vi "Path Keeper_User Find File.vi"(7 "Previous Path":path, 8 "error In":errorcluster, 9 "File(f)\nDirectory(t) In":bool, 11 "File / Directory Name In":string) -> (0 "error Out":errorcluster, 1 "Valid Item Out":bool, 3 "path Out":path)   [LabVIEW 2015]
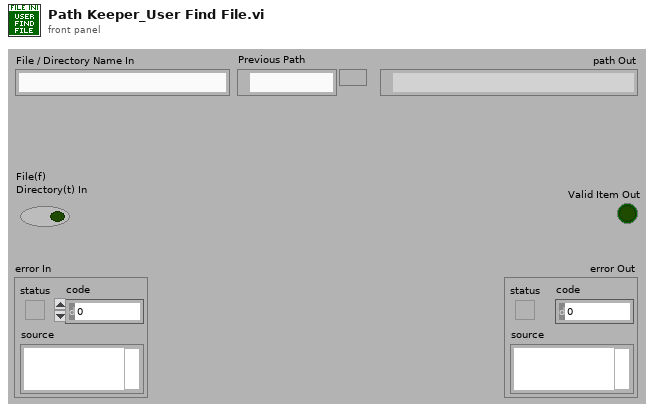
[diagram p1: front panel]
types:
  T1 = enum32{"existing file", "new file", "new or existing file", "existing dir", "new dir", "new or existing dir", "existing file (use LLBs)", "new file (use LLBs)", "new or existing file (use LLBs)", "new or existing file or directory (use LLBs)"}
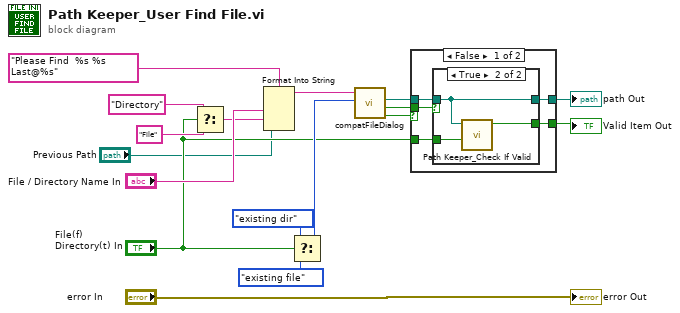
[diagram p0: block diagram]
diagram:
  n1 = Select(t="Directory" ("File / Directory Name In"), s="File(f)\nDirectory(t) In", f="File") -> (s? t:f=w6:string)
  n2 = Format Into String(format string="Please Find  %s %s Last@%s", "File / Directory Name In", w6, "Previous Path") -> (resulting string=w5:string)  [unwired: 2 in, 1 out]
  n3 = Select(t=T1."existing dir" ("select mode (2)"), s="File(f)\nDirectory(t) In", f=T1."existing file" ("select mode (2)")) -> (s? t:f=w13:T1)
  n4 = call <vilib>:"compatFileDialog.vi"("prompt"=w5, "select mode (2)"=w13) -> ("cancelled"=w16:bool, "exists"=w15:bool, "path"=w14:path)  [unwired: 7 in]
  n5 = case shown="False" w16 {
    tunnel: [w22 _] -> w17
    tunnel: w14 -> [w21 _]
    tunnel: w15 -> [w20 _]
    tunnel: [w19 _] -> w3
    tunnel: "File(f)\nDirectory(t) In" -> [w18 _]
    frame False {
      n6 = case shown="True" w20 {
        tunnel: [_ w25] -> w22
        tunnel: w21 -> [_ w24]
        tunnel: [_ w24] -> w19
        tunnel: w18 -> [_ w23]
        frame False {
        }
        frame True {
          n7 = call "Path Keeper_Check If Valid.vi"("File(f)\nDirectory(t) In"=w23, "path In"=w24) -> ("Valid Out"=w25:bool)  [unwired: 8 in, 1 out]
        }
      }
    }
    frame True {
    }
  }
  "Valid Item Out" <- w17
  "path Out" <- w3
  "error Out" <- "error In"
